vi "YMD log files.vi"(4 "Day":bool=TRUE, 5 "Month":bool=TRUE, 6 "Input text array":string[](array[string]), 7 "Input header array":string[](array[string]), 8 "Start new line":bool=TRUE, 9 "current time":timestamp, 10 "Log file name":string, 11 "Log file path":path) -> ()   [LabVIEW 2018]
panel:
  in  "Year":bool=TRUE
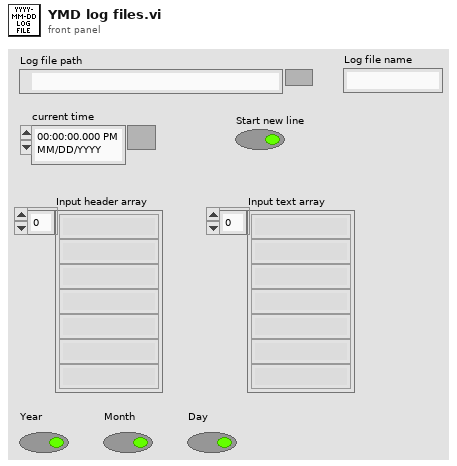
[diagram p1: front panel]
types:
  T1 = enum16{"open", "replace", "create", "open or create", "replace or create", "replace or create with confirmation"}
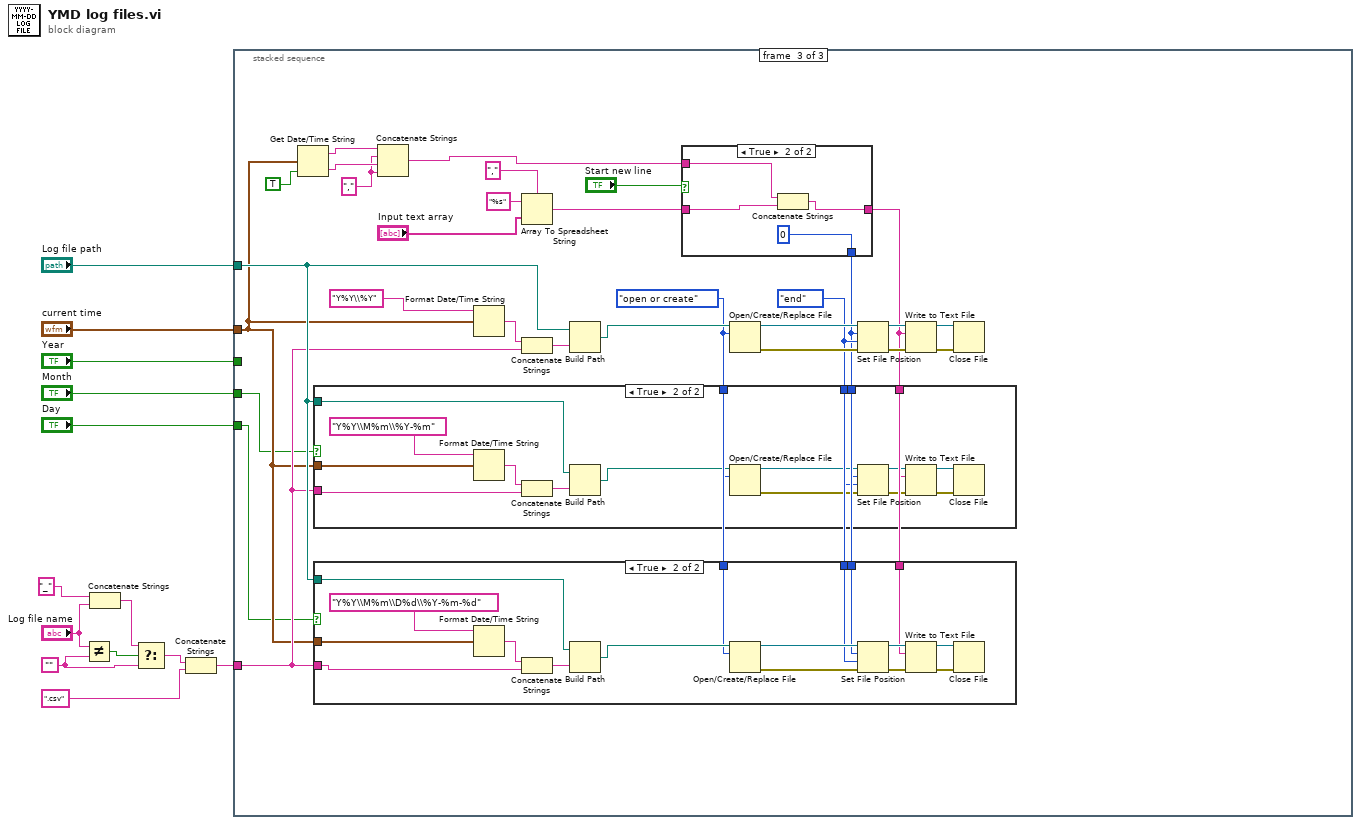
[diagram p0: block diagram]
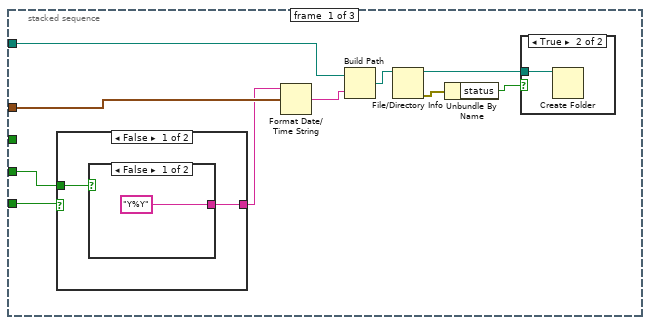
[diagram p2: hidden frame]
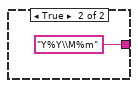
[diagram p3: hidden frame]
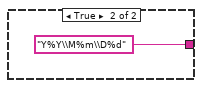
[diagram p4: hidden frame]
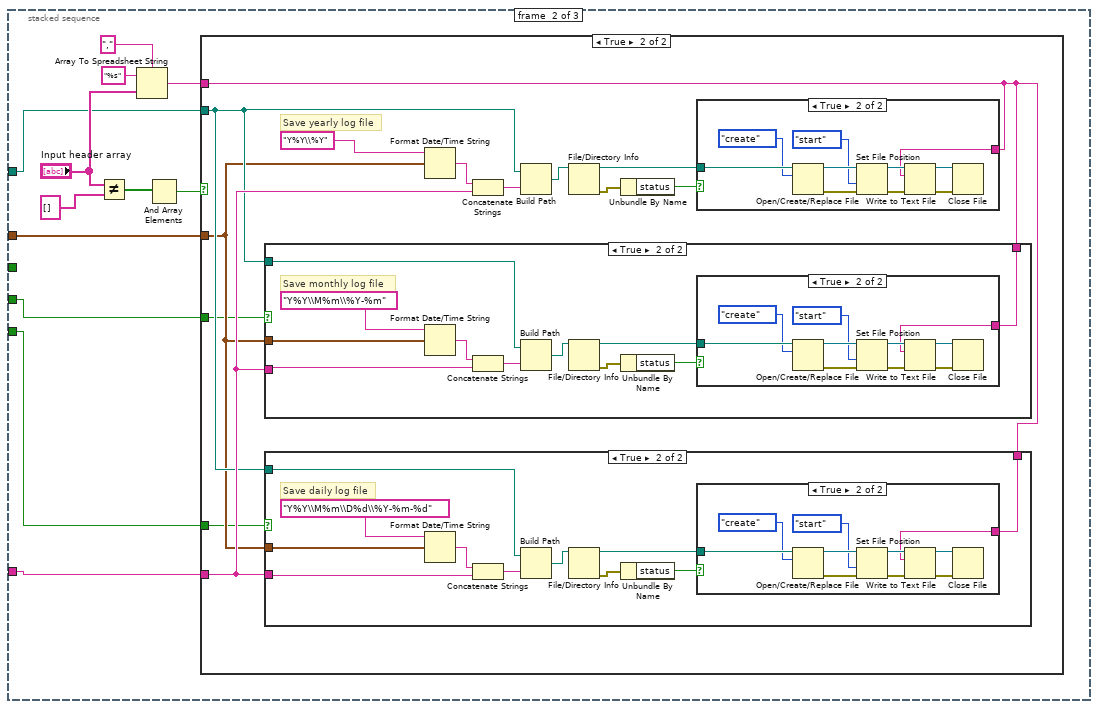
[diagram p6: hidden frame]
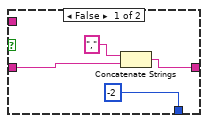
[diagram p15: hidden frame]
diagram:
  w8 = ""
  n1 = Not Equal?(x="Log file name", y=w8) -> (x != y?=w12:bool)
  n2 = Concatenate Strings("_" ("string"), "Log file name") -> (w9:string)
  n3 = Select(t=w9, s=w12, f=w8) -> (s? t:f=w7:string)
  n4 = Concatenate Strings(w7, ".csv" ("string")) -> (w6:string)
  n5 = stacked-sequence {
    tunnel: "current time" -> [w18 w32 w115]
    tunnel: "Log file path" -> [w17 w33 w123]
    tunnel: w6 -> [_ w35 w122]
    tunnel: "Day" -> [w16 w30 w108]
    tunnel: "Month" -> [w15 w31 w109]
    tunnel: "Year" -> [_ _ _]
    frame #0 {
      n6 = case shown="False" w16 {
        tunnel: w15 -> [w25 _]
        tunnel: [w24 "Y%Y\\M%m\\D%d" ("time format string (%c)")] -> w14
        frame False {
          n7 = case shown="False" w25 {
            tunnel: ["Y%Y" ("time format string (%c)") "Y%Y\\M%m" ("time format string (%c)")] -> w24
            frame False {
            }
            frame True {
            }
          }
        }
        frame True {
        }
      }
      n8 = Format Date/Time String(time format string (%c)=w14, seconds (now)=w18) -> (date/time string=w22:string)  [unwired: 1 out]
      n9 = Build Path(base path=w17, name or relative path=w22) -> (appended path=w23:path)
      n10 = File/Directory Info(path=w23) -> (path out=w19:path, error out=w21:errorcluster)  [unwired: 1 in, 5 out]
      n11 = Unbundle By Name(w21) -> ("status"=w20:bool)
      n12 = case shown="True" w20 {
        tunnel: w19 -> [_ w29]
        frame False {
        }
        frame True {
          n13 = Create Folder(path (use dialog)=w29) -> ()  [unwired: 1 in, 4 out]
        }
      }
    }
    frame #1 {
      n14 = Not Equal?(x="Input header array", y=string[] [] ("Input header array")) -> (x != y?=w40:bool[])
      n15 = Array To Spreadsheet String(delimiter (Tab)="," ("string"), array="Input header array", 3:"%s" ("format string")) -> (spreadsheet string=w34:string)
      n16 = And Array Elements(Boolean array=w40) -> (logical AND=w39:bool)
      n17 = case shown="True" w39 {
        tunnel: w35 -> [_ w47]
        tunnel: w34 -> [_ w46]
        tunnel: w33 -> [_ w45]
        tunnel: w32 -> [_ w44]
        tunnel: w31 -> [_ w43]
        tunnel: w30 -> [_ w42]
        frame False {
        }
        frame True {
          # "Save yearly log file"
          n18 = case shown="True" w43 {
            tunnel: w47 -> [_ w79]
            tunnel: w46 -> [_ w78]
            tunnel: w45 -> [_ w77]
            tunnel: w44 -> [_ w76]
            frame False {
            }
            frame True {
              # "Save monthly log file"
              n19 = Format Date/Time String(time format string (%c)="Y%Y\\M%m\\%Y-%m", seconds (now)=w76) -> (date/time string=w85:string)  [unwired: 1 out]
              n20 = Concatenate Strings(w85, w79) -> (w84:string)
              n21 = Build Path(base path=w77, name or relative path=w84) -> (appended path=w80:path)
              n22 = File/Directory Info(path=w80) -> (path out=w82:path, error out=w81:errorcluster)  [unwired: 1 in, 5 out]
              n23 = Unbundle By Name(w81) -> ("status"=w83:bool)
              n24 = case shown="True" w83 {
                tunnel: w82 -> [_ w96]
                tunnel: w78 -> [_ w87]
                frame False {
                }
                frame True {
                  n25 = Open/Create/Replace File(file path (use dialog)=w96, operation (0:open)=T1."create") -> (refnum out=w94:refnum<file>, error out=w93:errorcluster)  [unwired: 1 in, 4 out]
                  n26 = Set File Position(refnum=w94, from (0:start)=enum16{"start", "end", "current"}."start", error in=w93) -> (refnum out=w92:refnum<file>, error out=w95:errorcluster)  [unwired: 1 out]
                  n27 = Write to Text File(file (use dialog)=w92, text=w87, error in=w95) -> (refnum out=w91:refnum<file>, error out=w90:errorcluster)  [unwired: 2 out]
                  n28 = Close File(refnum=w91, error in=w90) -> ()  [unwired: 2 out]
                }
              }
            }
          }
          n29 = case shown="True" w42 {
            tunnel: w47 -> [_ w58]
            tunnel: w46 -> [_ w57]
            tunnel: w45 -> [_ w56]
            tunnel: w44 -> [_ w55]
            frame False {
            }
            frame True {
              # "Save daily log file"
              n30 = Format Date/Time String(time format string (%c)="Y%Y\\M%m\\D%d\\%Y-%m-%d", seconds (now)=w55) -> (date/time string=w64:string)  [unwired: 1 out]
              n31 = Concatenate Strings(w64, w58) -> (w63:string)
              n32 = Build Path(base path=w56, name or relative path=w63) -> (appended path=w59:path)
              n33 = File/Directory Info(path=w59) -> (path out=w61:path, error out=w60:errorcluster)  [unwired: 1 in, 5 out]
              n34 = Unbundle By Name(w60) -> ("status"=w62:bool)
              n35 = case shown="True" w62 {
                tunnel: w61 -> [_ w75]
                tunnel: w57 -> [_ w66]
                frame False {
                }
                frame True {
                  n36 = Open/Create/Replace File(file path (use dialog)=w75, operation (0:open)=T1."create") -> (refnum out=w73:refnum<file>, error out=w72:errorcluster)  [unwired: 1 in, 4 out]
                  n37 = Set File Position(refnum=w73, from (0:start)=enum16{"start", "end", "current"}."start", error in=w72) -> (refnum out=w71:refnum<file>, error out=w74:errorcluster)  [unwired: 1 out]
                  n38 = Write to Text File(file (use dialog)=w71, text=w66, error in=w74) -> (refnum out=w70:refnum<file>, error out=w69:errorcluster)  [unwired: 2 out]
                  n39 = Close File(refnum=w70, error in=w69) -> ()  [unwired: 2 out]
                }
              }
            }
          }
          n40 = Format Date/Time String(time format string (%c)="Y%Y\\%Y", seconds (now)=w44) -> (date/time string=w52:string)  [unwired: 1 out]
          n41 = Concatenate Strings(w52, w47) -> (w51:string)
          n42 = Build Path(base path=w45, name or relative path=w51) -> (appended path=w50:path)
          n43 = File/Directory Info(path=w50) -> (path out=w49:path, error out=w54:errorcluster)  [unwired: 1 in, 5 out]
          n44 = Unbundle By Name(w54) -> ("status"=w48:bool)
          n45 = case shown="True" w48 {
            tunnel: w49 -> [_ w106]
            tunnel: w46 -> [_ w97]
            frame False {
            }
            frame True {
              n46 = Open/Create/Replace File(file path (use dialog)=w106, operation (0:open)=T1."create") -> (refnum out=w104:refnum<file>, error out=w103:errorcluster)  [unwired: 1 in, 4 out]
              n47 = Set File Position(refnum=w104, from (0:start)=enum16{"start", "end", "current"}."start", error in=w103) -> (refnum out=w102:refnum<file>, error out=w105:errorcluster)  [unwired: 1 out]
              n48 = Write to Text File(file (use dialog)=w102, text=w97, error in=w105) -> (refnum out=w101:refnum<file>, error out=w100:errorcluster)  [unwired: 2 out]
              n49 = Close File(refnum=w101, error in=w100) -> ()  [unwired: 2 out]
            }
          }
        }
      }
    }
    frame #2 {
      w110 = "," ("string")
      w125 = T1."open or create" ("operation (0:open)")
      w124 = enum16{"start", "end", "current"}."end" ("from (0:start)")
      n50 = Get Date/Time String(seconds (now)=w115, want seconds? (F)=TRUE) -> (date string=w112:string, time string=w111:string)  [unwired: 1 out]
      n51 = Concatenate Strings(w112, w110, w111, w110) -> (w113:string)
      n52 = Format Date/Time String(time format string (%c)="Y%Y\\%Y", seconds (now)=w115) -> (date/time string=w134:string)  [unwired: 1 out]
      n53 = Array To Spreadsheet String(delimiter (Tab)="," ("string"), array="Input text array", 3:"%s" ("format string")) -> (spreadsheet string=w119:string)
      n54 = Concatenate Strings(w134, w122) -> (w135:string)
      n55 = Build Path(base path=w123, name or relative path=w135) -> (appended path=w126:path)
      n56 = case shown="True" "Start new line" {
        tunnel: [w171 w175] -> w118
        tunnel: w119 -> [w172 w176]
        tunnel: [i64 -2 ("offset (in bytes) (0)") i64 0 ("offset (in bytes) (0)")] -> w117
        tunnel: w113 -> [_ w174]
        frame False {
          n57 = Concatenate Strings("," ("string"), w172) -> (w171:string)
        }
        frame True {
          n58 = Concatenate Strings(w174, w176) -> (w175:string)
        }
      }
      n59 = case shown="True" w109 {
        tunnel: w125 -> [_ w142]
        tunnel: w124 -> [_ w141]
        tunnel: w123 -> [_ w140]
        tunnel: w122 -> [_ w139]
        tunnel: w118 -> [_ w138]
        tunnel: w117 -> [_ w137]
        tunnel: w115 -> [_ w136]
        frame False {
        }
        frame True {
          n60 = Format Date/Time String(time format string (%c)="Y%Y\\M%m\\%Y-%m", seconds (now)=w136) -> (date/time string=w151:string)  [unwired: 1 out]
          n61 = Concatenate Strings(w151, w139) -> (w152:string)
          n62 = Build Path(base path=w140, name or relative path=w152) -> (appended path=w150:path)
          n63 = Open/Create/Replace File(file path (use dialog)=w150, operation (0:open)=w142) -> (refnum out=w147:refnum<file>, error out=w146:errorcluster)  [unwired: 1 in, 4 out]
          n64 = Set File Position(offset (in bytes) (0)=w137, refnum=w147, from (0:start)=w141, error in=w146) -> (refnum out=w145:refnum<file>, error out=w148:errorcluster)
          n65 = Write to Text File(file (use dialog)=w145, text=w138, error in=w148) -> (refnum out=w144:refnum<file>, error out=w143:errorcluster)  [unwired: 2 out]
          n66 = Close File(refnum=w144, error in=w143) -> ()  [unwired: 2 out]
        }
      }
      n67 = case shown="True" w108 {
        tunnel: w125 -> [_ w162]
        tunnel: w124 -> [_ w161]
        tunnel: w123 -> [_ w157]
        tunnel: w122 -> [_ w156]
        tunnel: w118 -> [_ w155]
        tunnel: w117 -> [_ w154]
        tunnel: w115 -> [_ w153]
        frame False {
        }
        frame True {
          n68 = Format Date/Time String(time format string (%c)="Y%Y\\M%m\\D%d\\%Y-%m-%d", seconds (now)=w153) -> (date/time string=w168:string)  [unwired: 1 out]
          n69 = Concatenate Strings(w168, w156) -> (w169:string)
          n70 = Build Path(base path=w157, name or relative path=w169) -> (appended path=w163:path)
          n71 = Open/Create/Replace File(file path (use dialog)=w163, operation (0:open)=w162) -> (refnum out=w165:refnum<file>, error out=w160:errorcluster)  [unwired: 1 in, 4 out]
          n72 = Set File Position(offset (in bytes) (0)=w154, refnum=w165, from (0:start)=w161, error in=w160) -> (refnum out=w166:refnum<file>, error out=w159:errorcluster)
          n73 = Write to Text File(file (use dialog)=w166, text=w155, error in=w159) -> (refnum out=w167:refnum<file>, error out=w158:errorcluster)  [unwired: 2 out]
          n74 = Close File(refnum=w167, error in=w158) -> ()  [unwired: 2 out]
        }
      }
      n75 = Open/Create/Replace File(file path (use dialog)=w126, operation (0:open)=w125) -> (refnum out=w128:refnum<file>, error out=w129:errorcluster)  [unwired: 1 in, 4 out]
      n76 = Set File Position(offset (in bytes) (0)=w117, refnum=w128, from (0:start)=w124, error in=w129) -> (refnum out=w130:refnum<file>, error out=w127:errorcluster)
      n77 = Write to Text File(file (use dialog)=w130, text=w118, error in=w127) -> (refnum out=w131:refnum<file>, error out=w132:errorcluster)  [unwired: 2 out]
      n78 = Close File(refnum=w131, error in=w132) -> ()  [unwired: 2 out]
    }
  }
